vi "Check Filter Sw.vi"(8 "error in":errorcluster, 11 "CRDS in":refnum<class "CRDS.lvclass">) -> (0 "error out":errorcluster, 3 "CRDS out":refnum<class "CRDS.lvclass">)   [LabVIEW 2011, in "CRDS.lvclass"]
doc: "Check the filter switch duty cycle in the filter class (unless the filter cycle is overridden). This will set the <B>filter</B> shared variable to the value opposite of the current value stored in the Switch class. No other action is required as the Instrument will respond properly in the Rcv Cmd VI."
uses:
  CRDS.lvclass
  Reusable/Switch/Switch.lvclass
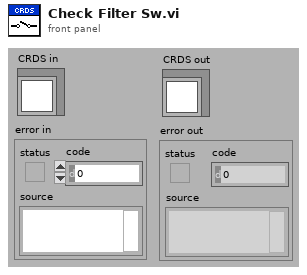
[diagram p1: front panel]
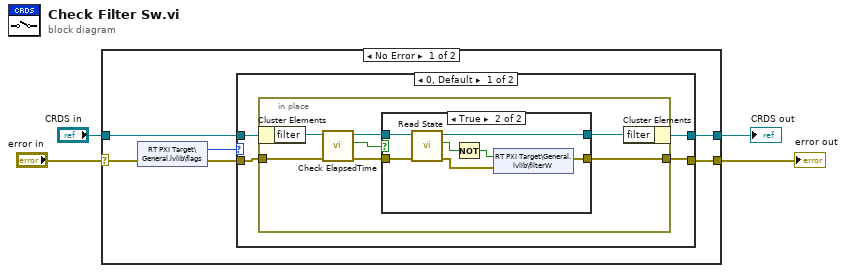
[diagram p0: block diagram]
diagram:
  n1 = case shown="No Error" "error in" {
    selector: "error in" -> [w6 w34]
    tunnel: [w9 w34] -> w3
    tunnel: [w8 w33] -> w1
    tunnel: "CRDS in" -> [w10 w33]
    frame No Error {
      n2 = shared-variable "RT PXI Target\\General.lvlib\\flags"(error in=w6) -> (w7:u8, error out=w5:errorcluster)
      n3 = case shown="0, Default" w7 {
        tunnel: w10 -> [w14 w32]
        tunnel: w5 -> [w13 w31]
        tunnel: [w12 w31] -> w9
        tunnel: [w11 w32] -> w8
        frame 0, Default {
          n4 = in-place {
            in-place-border: w13 -> [w20]
            in-place-border: [w17] -> w12
            n5 = in-place-cluster #1(w14) -> ("filter"=w21:refnum<class "Switch.lvclass">)
            n6 = call-dynamic "Check ElapsedTime.vi"("error in"=w20, "Switch in"=w21) -> ("error out"=w18:errorcluster, "TimeElapsed?"=w19:bool, "Switch out"=w16:refnum<class "Switch.lvclass">)  [unwired: 6 in, 1 out]
            n7 = case shown="True" w19 {
              tunnel: w18 -> [w23 w30]
              tunnel: [w23 w26] -> w17
              tunnel: w16 -> [w22 w29]
              tunnel: [w22 w27] -> w15
              frame False {
              }
              frame True {
                n8 = call-dynamic "Read State.vi"("error in (no error)"=w30, "Switch in"=w29) -> ("error out"=w28:errorcluster, "State"=w24:bool, "Switch out"=w27:refnum<class "Switch.lvclass">)  [unwired: 7 in]
                n9 = Not(x=w24) -> (.not. x?=w25:bool)
                n10 = shared-variable "RT PXI Target\\General.lvlib\\filterW"(w25, error in=w28) -> (error out=w26:errorcluster)
              }
            }
            n11 = in-place-cluster #1("filter"=w15) -> (w11:refnum<class "CRDS.lvclass">)
          }
        }
        frame 1 {
          # "Override filter duty cycle."
        }
      }
    }
    frame Error {
    }
  }
  "error out" <- w3
  "CRDS out" <- w1
